vi "Post Post Build Fixup.vi"() -> ()   [LabVIEW 2020]
uses:
  <vilib>/Utility/traverseref.llb/TRef TravTarget.ctl
  <vilib>/Utility/miscctls.llb/LVMapReplaceAction.ctl
  a8a67836-8e1b-4654-be25-c4f924580562.vi
  <vilib>/Utility/traverseref.llb/VI Scripting - Traverse.lvlib
panel:
  out "Deleting .vim from disk":path
  out "Disconnecting .vim from library":path
  out "Scanning VI...":path
  in  "Folder Path (Empty: Source Distrubution Built Folder)":path
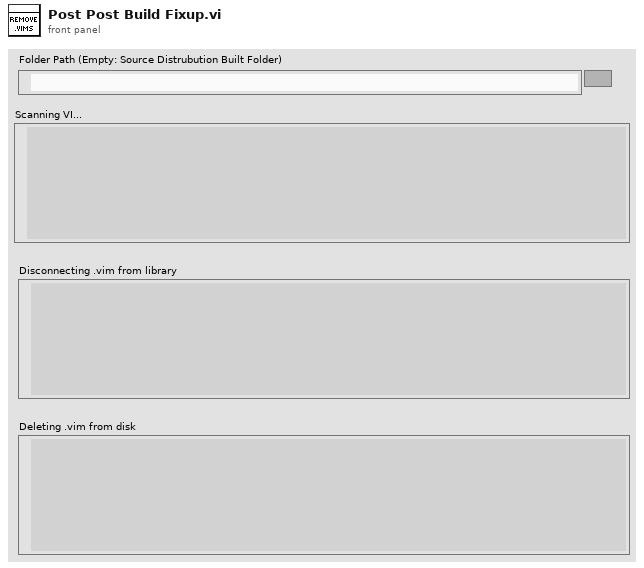
[diagram p1: front panel]
types:
  T1 = typedef "TRef TravTarget.ctl" = enum16{"FP", "BD", "Other"}
  T2 = typedef "LVMapReplaceAction.ctl" = enum32{"Modify Entry only if found", "Add or Modify Entry", "Delete Entry"}
  T3 = enum32{"Invalid", "Standard", "Closed", "Hidden", "Minimized", "Maximized"}
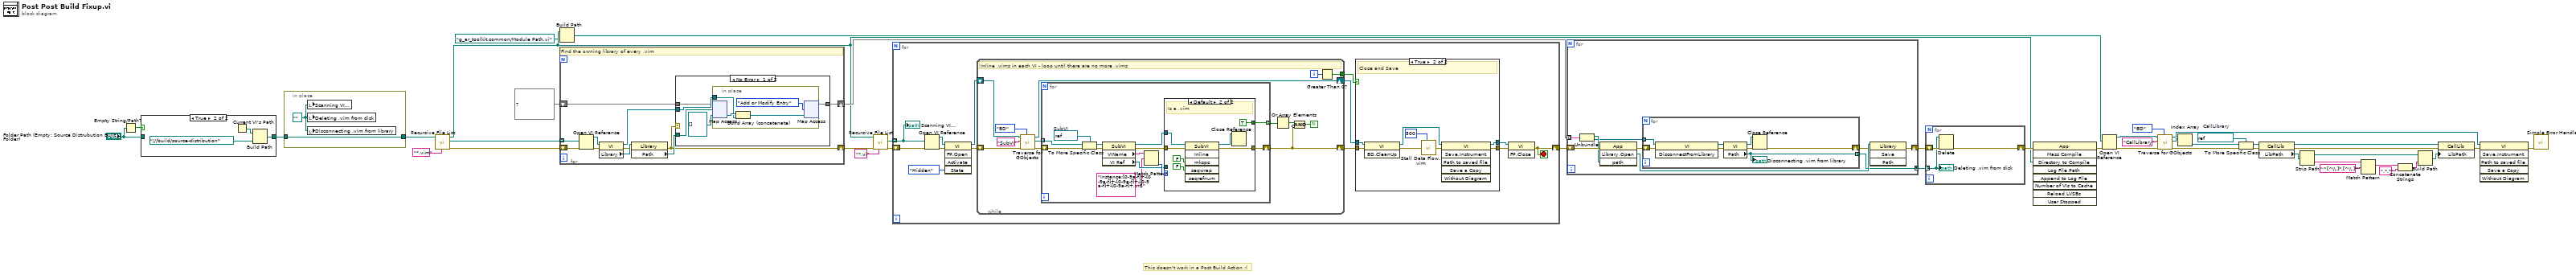
[diagram p0: block diagram]
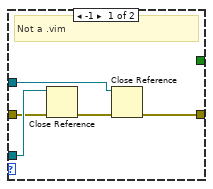
[diagram p3: hidden frame]
diagram:
  w17 = refnum<vi> refnum  # CallLibrary
  # "This doesn't work in a Post Build Action :("
  n1 = Empty String/Path?(string/path="Folder Path (Empty: Source Distrubution Built Folder)") -> (empty?=w30:bool)
  n2 = case shown="True" w30 {
    tunnel: [w45 w46] -> w29
    tunnel: "Folder Path (Empty: Source Distrubution Built Folder)" -> [w45 _]
    frame False {
    }
    frame True {
      n3 = Current VI's Path() -> (path=w48:path)
      n4 = Build Path(base path=w48, name or relative path=path "../../../build/source-distribution") -> (appended path=w46:path)
    }
  }
  n5 = in-place {
    in-place-border: [w49] -> w31
    in-place-border: w29 -> [w49]
    w50 = path "" ("Scanning VI...")
    n6 = local write "Scanning VI..."(w50) -> ()
    n7 = local write "Deleting .vim from disk"(w50) -> ()
    n8 = local write "Disconnecting .vim from library"(w50) -> ()
  }
  n9 = call <vilib>:"Recursive File List.vi"("pattern"="*.vim", "Folder Path"=w31) -> ("error out"=w42:errorcluster, "All Files in Dir"=w43:path[], "dup Folder Path"=w27:path)  [unwired: 5 in, 2 out]
  n10 = Build Path(base path=w27, name or relative path=path "g_ar_toolkit.common/Module Path.vi") -> (appended path=w24:path)
  n11 = for {
    tunnel: w43 -> [w58] mode=indexing
    shift-right: [w56] -> w35
    shift-left: map{path, refnum<vi>[]} {} ("Size: 0") -> [w55]
    shift-right: [w51] -> w40
    shift-left: w42 -> [w61]
    # "Find the owning library of every .vim"
    n12 = Open VI Reference(vi path=w58, error in (no error)=w61) -> (vi reference=w60:refnum<vi>, error out=w59:errorcluster)  [unwired: 4 in]
    n13 = property class="VI"(reference=w60, error in=w59) -> (reference out=w57:refnum<vi>, error out=w53:errorcluster, "Library"=w54:refnum<vi>)
    n14 = property class="Library"(reference=w54, error in=w53) -> (error out=w51:errorcluster, "Path"=w52:path)  [unwired: 1 out]
    n15 = case shown="No Error" w51 {
      tunnel: w57 -> [w66 _]
      tunnel: [w64 w71] -> w56
      tunnel: w55 -> [w63 w71]
      tunnel: w52 -> [w62 _]
      frame No Error {
        n16 = in-place {
          in-place-border: w66 -> [w68]
          n17 = in-place-map #1(w63, w62, refnum<vi>[] []) -> (w70:refnum<vi>[])  [unwired: 1 out]
          n18 = Build Array (concatenate)(w70, w68) -> (w67:refnum<vi>[])
          n19 = in-place-map #1(w67, LVMapReplaceAction."Add or Modify Entry" ("action")) -> (w64:map{path, refnum<vi>[]})  [unwired: 2 out]
        }
      }
      frame Error {
      }
    }
  }
  n20 = call <vilib>:"Recursive File List.vi"("pattern"="*.vi", "error in (no error)"=w40, "Folder Path"=w27) -> ("error out"=w38:errorcluster, "All Files in Dir"=w37:path[])  [unwired: 4 in, 3 out]
  n21 = for {
    shift-right: [w72] -> w36
    shift-left: w38 -> [w80]
    tunnel: w37 -> [w78] mode=indexing
    stop <- w72 stop-if-true
    n22 = Open VI Reference(vi path=w78, error in (no error)=w80) -> (vi reference=w74:refnum<vi>, error out=w79:errorcluster)  [unwired: 4 in]
    n23 = invoke class="VI" method="FP.Open"(reference=w74, error in=w79, "State"=T3."Hidden") -> (reference out=w81:refnum<vi>, error out=w73:errorcluster)  [unwired: 2 in, 3 out]
    n24 = while {
      shift-right: [w95] -> w76
      shift-left: w81 -> [w96]
      shift-right: [w85] -> w83
      shift-left: w73 -> [w94]
      tunnel: [w88] -> w77
      i -> [w89]
      stop <- w86 continue-if-true
      # "Inline .vims in each VI - loop until there are no more .vims"
      n25 = call <vilib>:"Traverse for GObjects.vi"("Traverse Target"=TRef_TravTarget."BD", "error in (no error)"=w94, "Class Name"="SubVI", "VI Refnum"=w96) -> ("error out"=w93:errorcluster, "References"=w91:refnum<vi>[], "dup VI Refnum"=w95:refnum<vi>)  [unwired: 4 in, 1 out]
      n26 = for {
        shift-right: [w104] -> w85
        shift-left: w93 -> [w110]
        tunnel: w91 -> [w109] mode=indexing
        tunnel: [w103] -> w97 mode=indexing
        w108 = refnum<vi> refnum  # SubVI
        n27 = To More Specific Class(target class=w108, reference=w109, error in=w110) -> (specific class reference=w107:refnum<vi>, error out=w106:errorcluster)
        n28 = property class="SubVI"(reference=w107, error in=w106) -> (reference out=w99:refnum<vi>, error out=w102:errorcluster, "VIName"=w105:string, "VI Ref"=w100:refnum<vi>)
        n29 = Match Pattern(string=w105, regular expression="Instance:[0-9a-f]+-[0-9a-f]+-[0-9a-f]+-[0-9a-f]+-[0-9a-f]+.vi$") -> (offset past match=w101:i32)  [unwired: 1 in, 3 out]
        n30 = case shown="Default" w101 {
          tunnel: [w115 w122] -> w104
          tunnel: w100 -> [w113 _]
          tunnel: [_ TRUE] -> w103
          tunnel: w102 -> [w111 w117]
          tunnel: w99 -> [w114 w120]
          frame -1 {
            # "Not a .vim"
            n31 = Close Reference(reference=w113, error in (no error)=w111) -> (error out=w112:errorcluster)
            n32 = Close Reference(reference=w114, error in (no error)=w112) -> (error out=w115:errorcluster)
          }
          frame Default {
            # "Is a .vim"
            n33 = invoke class="SubVI" method="Inline"(reference=w120, error in=w117, "mkspc"=FALSE ("Make Space in Block Diagram"), "seqwrap"=FALSE ("Wrap in Sequence")) -> (reference out=w116:refnum<vi>, error out=w122:errorcluster)  [unwired: 2 in, 4 out]
            n34 = Close Reference(reference=w116) -> ()  [unwired: 1 in, 1 out]
          }
        }
      }
      n35 = Or Array Elements(Boolean array=w97) -> (logical OR=w90:bool)
      n36 = Compound Arithmetic op=AND(w90, invert w85) -> (w86:bool)
      n37 = Greater Than 0?(x=w89) -> (x > 0?=w88:bool)
    }
    n38 = case shown="True" w77 {
      tunnel: w76 -> [w123 w132]
      tunnel: w83 -> [w124 w131]
      tunnel: [w124 w128] -> w82
      tunnel: [w123 w127] -> w75
      frame False {
        # "No Updates"
      }
      frame True {
        # "Close and Save"
        n39 = invoke class="VI" method="BD.CleanUp"(reference=w132, error in=w131) -> (reference out=w130:refnum<vi>, error out=w129:errorcluster)  [unwired: 1 in, 1 out]
        n40 = call "Stall Data Flow.vim"("value in"=w129, "milliseconds to wait"=u32 500) -> ("value out"=w126:errorcluster)  [unwired: 1 out]
        n41 = invoke class="VI" method="Save.Instrument"(reference=w130, error in=w126) -> (reference out=w127:refnum<vi>, error out=w128:errorcluster)  [unwired: 4 in, 4 out]
      }
    }
    n42 = invoke class="VI" method="FP.Close"(reference=w75, error in=w82) -> (error out=w72:errorcluster)  [unwired: 1 in, 2 out]
    "Scanning VI..." <- w78
  }
  n43 = for {
    shift-right: [w134] -> w33
    shift-left: w36 -> [w140]
    tunnel: w35 -> [w141] mode=indexing
    tunnel: [w133] -> w34 mode=concatenating
    n44 = Unbundle(w141) -> ("Library"=w139:path, w137:refnum<vi>[])
    n45 = invoke class="App" method="Library.Open"(error in=w140, "path"=w139) -> (error out=w138:errorcluster, "Open Library"=w136:refnum<vi>)  [unwired: 2 in, 2 out]
    n46 = for {
      shift-right: [w144] -> w135
      shift-left: w138 -> [w148]
      tunnel: w137 -> [w149] mode=indexing
      tunnel: [w142] -> w133 mode=indexing
      n47 = invoke class="VI" method="DisconnectFromLibrary"(reference=w149, error in=w148) -> (reference out=w146:refnum<vi>, error out=w147:errorcluster)  [unwired: 1 in, 1 out]
      n48 = property class="VI"(reference=w146, error in=w147) -> (reference out=w143:refnum<vi>, error out=w145:errorcluster, "Path"=w142:path)
      "Disconnecting .vim from library" <- w142
      n49 = Close Reference(reference=w143, error in (no error)=w145) -> (error out=w144:errorcluster)
    }
    n50 = invoke class="Library" method="Save"(reference=w136, error in=w135) -> (error out=w134:errorcluster)  [unwired: 2 in, 3 out]
  }
  n51 = for {
    tunnel: w34 -> [w150] mode=indexing
    shift-right: [w151] -> w32
    shift-left: w33 -> [w152]
    n52 = Delete(path (use dialog)=w150, error in=w152) -> (error out=w151:errorcluster)  [unwired: 3 in, 2 out]
    "Deleting .vim from disk" <- w150
  }
  n53 = invoke class="App" method="Mass Compile"(error in=w32, "Directory to Compile"=w27) -> (error out=w25:errorcluster)  [unwired: 7 in, 8 out]
  n54 = Open VI Reference(vi path=w24, error in (no error)=w25) -> (vi reference=w22:refnum<vi>, error out=w23:errorcluster)  [unwired: 4 in]
  n55 = call <vilib>:"Traverse for GObjects.vi"("Traverse Target"=TRef_TravTarget."BD", "error in (no error)"=w23, "Class Name"="CallLibrary", "VI Refnum"=w22) -> ("error out"=w16:errorcluster, "References"=w19:refnum<vi>[], "dup VI Refnum"=w2:refnum<vi>)  [unwired: 4 in, 1 out]
  n56 = Index Array(array=w19) -> (element=w18:refnum<vi>)  [unwired: 1 in]
  n57 = To More Specific Class(target class=w17, reference=w18, error in=w16) -> (specific class reference=w15:refnum<vi>, error out=w14:errorcluster)
  n58 = property class="CallLib"(reference=w15, error in=w14) -> (reference out=w5:refnum<vi>, error out=w6:errorcluster, "LibPath"=w13:path)
  n59 = Strip Path(path=w13) -> (stripped path=w12:path, name=w11:string)
  n60 = Match Pattern(string=w11, regular expression="^[^\\.]*.[^\\.]*") -> (match substring=w9:string)  [unwired: 1 in, 3 out]
  n61 = Concatenate Strings(w9, ".*.*" ("string")) -> (w7:string)
  n62 = Build Path(base path=w12, name or relative path=w7) -> (appended path=w4:path)
  n63 = property class="CallLib"(reference=w5, error in=w6, "LibPath"=w4) -> (error out=w3:errorcluster)  [unwired: 1 out]
  n64 = invoke class="VI" method="Save.Instrument"(reference=w2, error in=w3) -> (error out=w1:errorcluster)  [unwired: 4 in, 5 out]
  n65 = call <vilib>:"Simple Error Handler.vi"("error in (no error)"=w1) -> ()  [unwired: 4 in, 5 out]
